vi "Open RFSG.vi"(8 "error in":errorcluster {"code" format="%.0x"}, 9 "Bitfile":string="DriverSetup=Bitfile:niVSTFPGA_UART.lvbitx", 10 "Clock Source":T1="OnboardClock", 11 "Resource Name":refnum<k15>="PXI1Slot11") -> (0 "error out":errorcluster, 3 "IVI Refnum out":refnum<k15>)   [LabVIEW 2018]
uses:
  <instrlib>/niRFSG/niRFSG.llb/niRFSG Ref Clock Sources.ctl
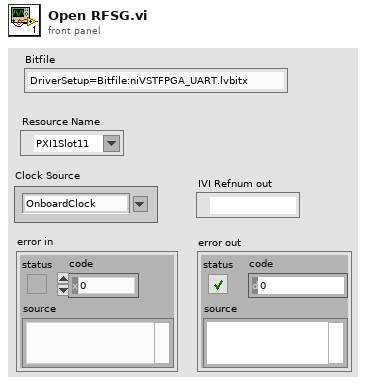
[diagram p1: front panel]
types:
  T1 = typedef "niRFSG Ref Clock Sources.ctl" = string
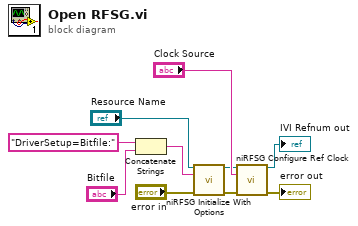
[diagram p0: block diagram]
diagram:
  n1 = Concatenate Strings("DriverSetup=Bitfile:" ("string"), "Bitfile") -> (w1:string)
  n2 = call <instrlib>:"niRFSG Initialize With Options.vi"("resource name"="Resource Name", "option string"=w1, "error in"="error in") -> ("instrument handle"=w6:refnum<k15>, "error out"=w7:errorcluster)  [unwired: 11 in]
  n3 = call <instrlib>:"niRFSG Configure Ref Clock.vi"("instrument handle"=w6, "ref clock source"="Clock Source", "error in"=w7) -> ("instrument handle out"=→"IVI Refnum out":refnum<k15>, "error out"=→"error out":errorcluster)  [unwired: 11 in]
